vi "FGV.vi"(1 "error in (no error)":errorcluster caption="에러 입력(에러 없음)", 3 "In":dbl, 4 "상태 컨트롤":enum16{"초기화", "읽기", "쓰기"}(ring)) -> (0 "error out":errorcluster caption="에러 출력", 2 "Out":dbl)   [LabVIEW 2018]
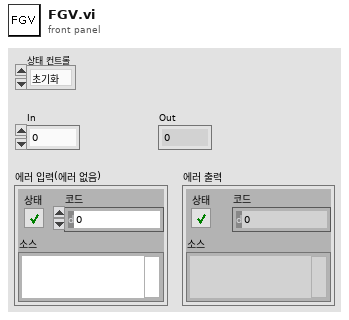
[diagram p1: front panel]
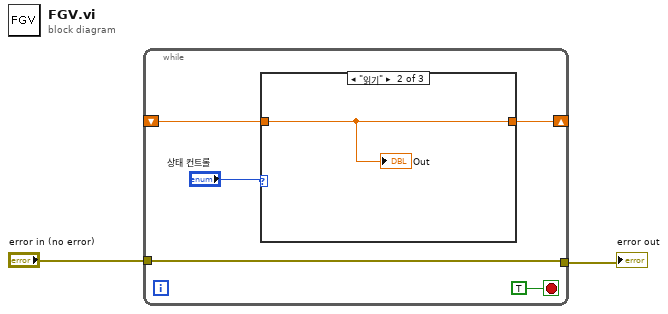
[diagram p0: block diagram]
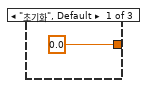
[diagram p2: hidden frame]
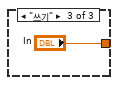
[diagram p3: hidden frame]
diagram:
  n1 = while {
    shift-right: [w6] -> _
    shift-left: _ -> [w4]
    tunnel: "error in (no error)" -> [w3]
    tunnel: [w3] -> w1
    stop <- TRUE stop-if-true
    n2 = case shown="\"읽기\"" "상태 컨트롤" {
      tunnel: [0.0 w9 "In"] -> w6
      tunnel: w4 -> [_ w9 _]
      frame "초기화", Default {
      }
      frame "읽기" {
        "Out" <- w9
      }
      frame "쓰기" {
      }
    }
  }
  "error out" <- w1
